vi "PlayerInit.vi"(8 "Default Positions":i16[](array[numeric])=[0], 9 "Filename":string, 11 "NXT":T1={"Hardware"="NXT", "Flattened String"=""}) -> (3 "NXT":T1={"Hardware"="NXT", "Flattened String"=""})   [LabVIEW 2010, in "Player.lvlib"]
uses:
  Player.lvlib
  <vilib>/NXT/Subs/LVHSConnector.ctl
  Components/Components.lvlib
  Timer Extensions/timerExts.lvlib
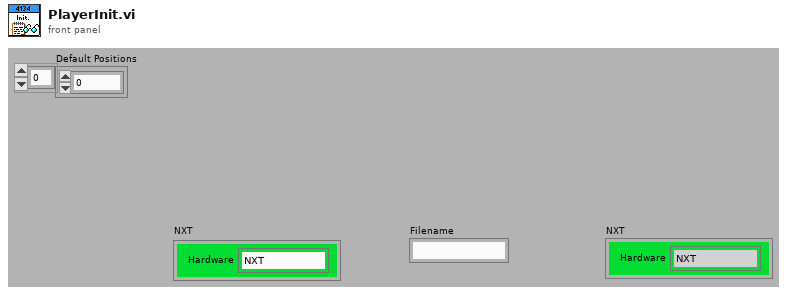
[diagram p1: front panel]
types:
  T1 = typedef "LVHSConnector.ctl" = cluster{"Hardware":string, "Flattened String":string}
  T2 = typedef "timerExts.lvlib/Branched Timer.ctl" = cluster{"Type":enum8{"Branched Timer", "NXT Timer"}, "Index":u16}
  T3 = typedef "NXT_FileStatusCodes.ctl" = u16
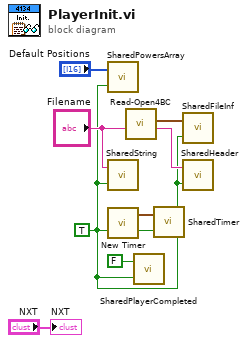
[diagram p0: block diagram]
diagram:
  w1 = TRUE ("Write?")
  n1 = call "SharedPowersArray.vi"("Write?"=w1, "PowersInput"="Default Positions") -> ()  [unwired: 1 out]
  n2 = call "SharedString.vi"("Write?"=w1, "StringInput"="Filename") -> ()  [unwired: 1 out]
  n3 = call "New Timer.vi"() -> ("Branched Timer Index"=w2:T2)  [unwired: 4 in]
  n4 = call "Read-Open4BC.vi"("File"="Filename") -> ("Header"=w5:string, "File Information"=w3:cluster{"File Handle Out":u8, "Error out":T3})  [unwired: 7 in, 2 out]
  n5 = call "SharedPlayerCompleted.vi"("Write?"=w1, "PlayerCompletedInput"=FALSE) -> ()  [unwired: 1 out]
  n6 = call "SharedTimer.vi"("Write?"=w1, "TimerInput"=w2) -> ()  [unwired: 1 out]
  n7 = call "SharedFileInf.vi"("Write?"=w1, "FileInfInput"=w3) -> ()  [unwired: 1 out]
  n8 = call "SharedHeader.vi"("Write?"=w1, "HeaderInput"=w5) -> ()  [unwired: 1 out]
  "NXT" <- "NXT"
